vi "Untitled 2 (SubVI).vi"(4 "dt (ms)":u32, 5 "Kp":dbl, 6 "Omega":dbl, 7 "Td":dbl, 8 "Reference":dbl, 9 "E(n-1)":dbl, 10 "I(n-1)":dbl, 11 "Ti":dbl) -> (1 "u":dbl, 2 "E(n)":dbl, 3 "I(n)":dbl)   [LabVIEW 2016]
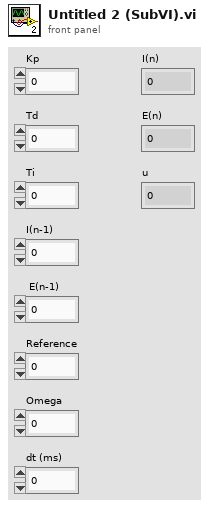
[diagram p1: front panel]
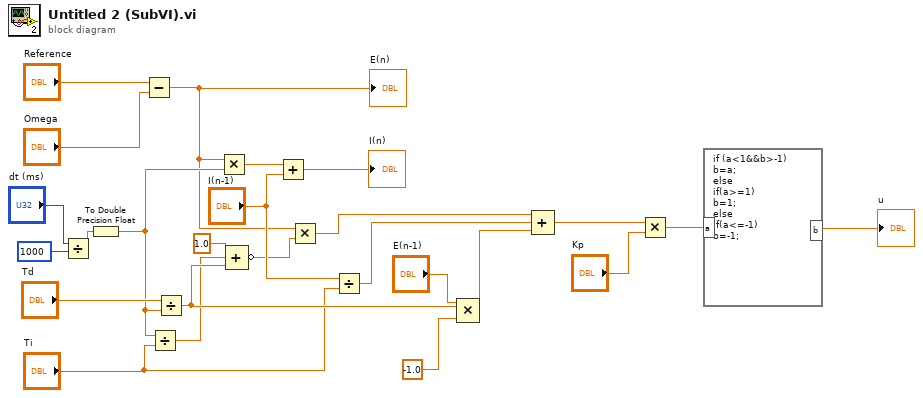
[diagram p0: block diagram]
diagram:
  n1 = Divide(x="dt (ms)", y=u32 1000) -> (x/y=w3:dbl)
  n2 = To Double Precision Float(number=w3) -> (double precision float=w6:dbl)
  n3 = Subtract(x="Reference", y="Omega") -> (x-y=w4:dbl)
  "E(n)" <- w4
  n4 = Divide(x=w6, y="Ti") -> (x/y=w15:dbl)
  n5 = Divide(x="Td", y=w6) -> (x/y=w21:dbl)
  n6 = Multiply(x=w4, y=w6) -> (x*y=w8:dbl)
  n7 = Compound Arithmetic op=ADD(1.0 ("value"), w15, w21) -> (invert w5:dbl)
  n8 = Add(x=w8, y="I(n-1)") -> (x+y=→"I(n)":dbl)
  n9 = Multiply(x=w4, y=w5) -> (x*y=w12:dbl)
  n10 = Divide(x="I(n-1)", y="Ti") -> (x/y=w19:dbl)
  n11 = Compound Arithmetic op=MULTIPLY("E(n-1)", w21, -1.0 ("value")) -> (w23:dbl)
  n12 = Compound Arithmetic op=ADD(w12, w19, w23) -> (w24:dbl)
  n13 = Multiply(x=w24, y="Kp") -> (x*y=w9:dbl)
  n14 = formula code="if (a<1&&b>-1)\nb=a;\nelse \nif(a>=1)\nb=1;\nelse\nif(a<=-1)\nb=-1;"("a"=w9) -> ("b"=→"u":dbl)
